vi "closeOutput.vi"(8 "error in (no error)":errorcluster, 11 "DIO64Output in":refnum<class "DIO64Output.lvclass">) -> (0 "error out":errorcluster)   [LabVIEW 2009, in "Hardware.lvlib" / "Channels.lvlib" / "DIO64Output.lvclass"]
uses:
  DIO64Output.lvclass
  DIO64Output.lvclass/DIO64Output.ctl
  Channels.lvlib
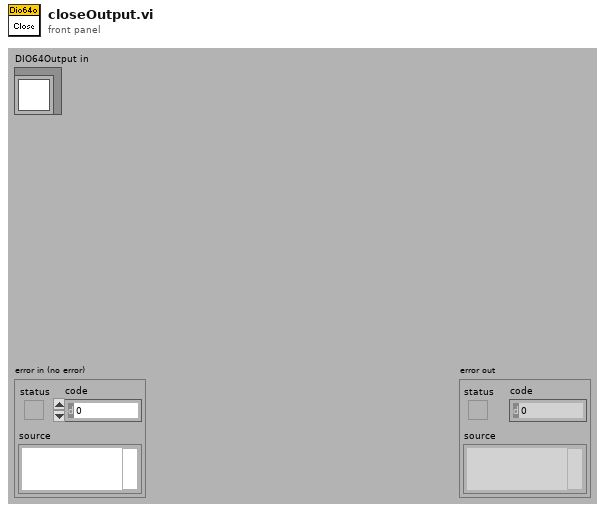
[diagram p1: front panel]
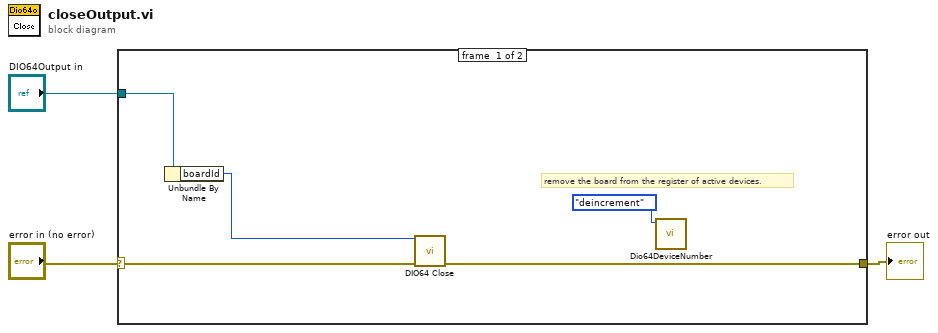
[diagram p0: block diagram]
diagram:
  n1 = case shown="No Error" "error in (no error)" {
    selector: "error in (no error)" -> [w4 w9]
    tunnel: "DIO64Output in" -> [w6 _]
    tunnel: [w7 w9] -> w1
    frame #0 {
      # "remove the board from the register of active devices."
      n2 = Unbundle By Name(w6) -> ("boardId"=w5:i32)
      n3 = call <userlib>:"DIO64 Close.vi"("board in"=w5, "error in (no error)"=w4) -> ("error out"=w7:errorcluster)  [unwired: 12 in, 1 out]
      n4 = call "Dio64DeviceNumber.vi"("Action"=enum16{"increment", "deincrement"}."deincrement") -> ()  [unwired: 10 in, 1 out]
    }
    frame #1 {
    }
  }
  "error out" <- w1
